vi "create folder.vi"(9 "Parent":refnum<class "system object.lvclass">, 10 "name":string) -> (3 "Folder.lvclass":refnum<class "Folder.lvclass">)   [LabVIEW 2020, in "Folder.lvclass"]
uses:
  Folder.lvclass
  Folder.lvclass/Folder.ctl
  system object/system object.lvclass
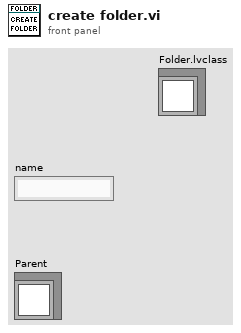
[diagram p1: front panel]
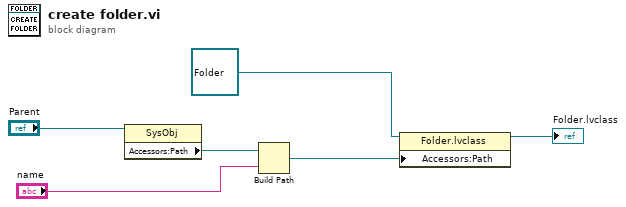
[diagram p0: block diagram]
diagram:
  n1 = property class="SysObj"(reference="Parent") -> ("Accessors:Path"=w3:path)  [unwired: 1 in, 2 out]
  n2 = Build Path(base path=w3, name or relative path="name") -> (appended path=w1:path)
  n3 = property class="Folder.lvclass"(reference=refnum<class "Folder.lvclass"> refnum ("Folder.lvclass 2"), "Accessors:Path"=w1) -> (reference out=→"Folder.lvclass":refnum<class "Folder.lvclass">)  [unwired: 1 in, 1 out]
